vi "VScaleInfo.vi"() -> (0 "Voltage Scale":T1, 1 "Total Gain (dB)":dbl, 2 "Dig Word Size":u16, 4 "vGain scalar":dbl)   [LabVIEW 2015]
uses:
  ScanSystem.llb/MotionGlobals.vi
  <instrlib>/Acqiris Dx/Acqiris Dx.lvlib
  <instrlib>/Acqiris Bx/Acqiris Bx.lvlib
panel:
  out "vGain (dB)":dbl
  in  "Channel (1)":i32=1
  in  "Instrument ID":u32
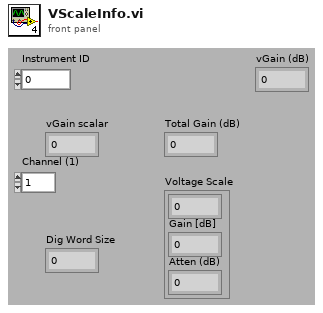
[diagram p1: front panel]
types:
  T1 = cluster{dbl, "Gain [dB]  ":dbl, "Atten (dB)":sgl}
  T2 = typedef "pulser.ctl" = enum16{"Pan 5900", "Agilent 33xxx", "WMC Mono-Cycle", "No Pulser", "NYU AVTECH", "Tabor W1281A", "Daxsonics BP1", "Pan 5800", "Daxsonics BP2"}
  T3 = cluster{"Energy (microJ)":u8, "Damping (In Ohm)":u8, "HP Filt(KHz) ":u8, "LP Filt (MHz)":u8, "Gain (db)":u8, "Atten (dB)":sgl}
  T4 = cluster{"Full Scale":dbl, "Gain [dB]  ":dbl, "Atten (dB)":sgl}
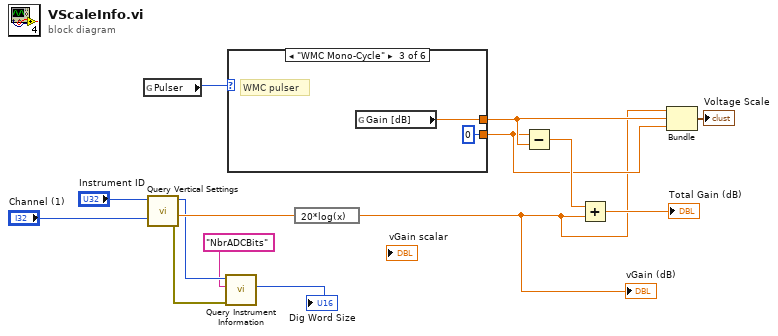
[diagram p0: block diagram]
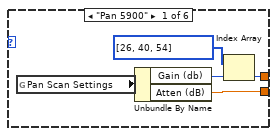
[diagram p2: hidden frame]
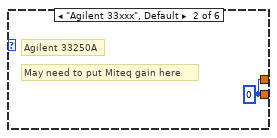
[diagram p3: hidden frame]
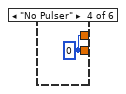
[diagram p4: hidden frame]
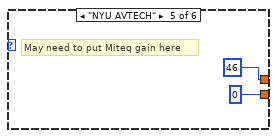
[diagram p5: hidden frame]
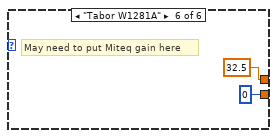
[diagram p6: hidden frame]
diagram:
  n1 = global read "MotionGlobals.vi" "Pulser"() -> (w9:T2)
  n2 = call <instrlib>:"Query Vertical Settings.vi"("Instrument ID"="Instrument ID", "Channel (1)"="Channel (1)") -> ("dup Instrument ID"=w4:u32, "Full Scale"=w6:dbl, "error out"=w3:errorcluster)  [unwired: 1 in, 4 out]
  n3 = call <instrlib>:"Query Instrument Information.vi"("Instrument ID"=w4, "Parameter String"="NbrADCBits", "error in (no error)"=w3) -> ("Info Value (I32)"=→"Dig Word Size":i32)  [unwired: 1 in, 5 out]
  n4 = case shown="\"WMC Mono-Cycle\"" w9 {
    tunnel: [w16 w20 0 w23 0 0] -> w10
    tunnel: [w15 w20 w22 w23 46 32.5] -> w11
    frame "Pan 5900" {
      n5 = global read "MotionGlobals.vi" "Pan Scan Settings"() -> (w17:T3)
      n6 = Unbundle By Name(w17) -> ("Gain (db)"=w19:u8, "Atten (dB)"=w16:sgl)
      n7 = Index Array(array=i32[] [26, 40, 54], index=w19) -> (element=w15:i32)
    }
    frame "Agilent 33xxx", Default {
      w20 = 0
      # "Agilent 33250A"
      # "May need to put Miteq gain here"
    }
    frame "WMC Mono-Cycle" {
      # "WMC pulser"
      n8 = global read "MotionGlobals.vi" "Gain [dB]"() -> (w22:sgl)
    }
    frame "No Pulser" {
      w23 = 0
    }
    frame "NYU AVTECH" {
      # "May need to put Miteq gain here"
    }
    frame "Tabor W1281A" {
      # "May need to put Miteq gain here"
    }
  }
  n9 = expression code="20*log(x)"(w6) -> (w5:dbl)
  "vGain (dB)" <- w5
  n10 = Subtract(x=w10, y=w11) -> (x-y=w13:dbl)
  n11 = Add(x=w13, y=w5) -> (x+y=→"Total Gain (dB)":dbl)
  n12 = Bundle("Full Scale"=w5, "Gain [dB]"=w11, "Atten (dB)"=w10) -> (→"Voltage Scale":T4)  [unwired: 1 out]
